vi "Write Outlet Temp.vi"(0 "Line":tag="Dev1/port0/line0:7", 5 "Outlet Temp":dbl, 11 "Error In":errorcluster) -> (15 "Error Out":errorcluster)   [LabVIEW 2014]
doc: "This VI generates a static analog voltage output on the line you specify."
uses:
  <vilib>/DAQmx/create/channels.llb/DAQmx Create Channel (AO-Voltage-Basic).vi
  <vilib>/DAQmx/write.llb/DAQmx Write (Analog DBL 1Chan 1Samp).vi
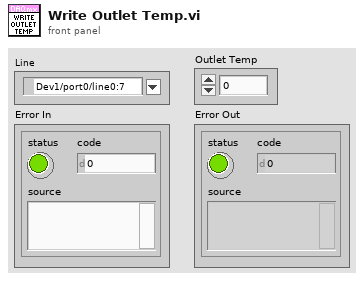
[diagram p1: front panel]
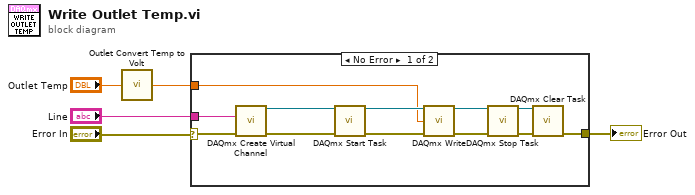
[diagram p0: block diagram]
diagram:
  n1 = call "Outlet Convert Temp to Volt.vi"("Outlet Temperature"="Outlet Temp") -> ("Outlet Voltage"=w1:dbl)
  n2 = case shown="No Error" "Error In" {
    selector: "Error In" -> [w9 w18]
    tunnel: "Line" -> [w8 _]
    tunnel: w1 -> [w7 _]
    tunnel: [w6 w18] -> w3
    frame No Error {
      n3 = call-poly <vilib>:"DAQmx Create Virtual Channel.vi"("physical channels"=w8, "error in"=w9) -> ("task out"=w14:refnum<k21>, "error out"=w15:errorcluster)  [unwired: 12 in]
      n4 = call <vilib>:"DAQmx Start Task.vi"("task/channels in"=w14, "error in"=w15) -> ("task out"=w17:refnum<k21>, "error out"=w16:errorcluster)  [unwired: 12 in]
      n5 = call-poly <vilib>:"DAQmx Write.vi"("task/channels in"=w17, "data"=w7, "error in"=w16) -> ("task out"=w11:refnum<k21>, "error out"=w10:errorcluster)  [unwired: 10 in, 1 out]
      n6 = call <vilib>:"DAQmx Stop Task.vi"("task/channels in"=w11, "error in"=w10) -> ("task out"=w13:refnum<k21>, "error out"=w12:errorcluster)  [unwired: 12 in]
      n7 = call <vilib>:"DAQmx Clear Task.vi"("task in"=w13, "error in"=w12) -> ("error out"=w6:errorcluster)  [unwired: 13 in]
    }
    frame Error {
    }
  }
  "Error Out" <- w3
